vi "get mapped channels.vi"(7 "owner":string, 11 "engine configuration in":refnum<class "engine configuration.lvclass">) -> (1 "write channels":refnum<class "TBM channel.lvclass">[](array[class]), 2 "read channels":refnum<class "TBM channel.lvclass">[](array[class]), 3 "engine configuration out":refnum<class "engine configuration.lvclass">, 4 "paired read tag":refnum<class "tag descriptor.lvclass">[](array[class]), 6 "paired write tag":refnum<class "tag descriptor.lvclass">[](array[class]))   [LabVIEW 2013, in "engine configuration.lvclass"]
doc: "This function returns the list of the owner's read and write channels that have been mapped to tags."
uses:
  engine configuration.lvclass
  <vilib>/NI/Tag Bus Module Framework/channel/TBM channel.lvclass
  <vilib>/NI/Tag Bus/tag/tag descriptor.lvclass
  engine configuration.lvclass/engine configuration.ctl
  <vilib>/NI/Tag Bus/tag/tag descriptor.lvclass/tag descriptor.ctl
  <vilib>/NI/Tag Bus Module Framework/channel/channel classification.ctl
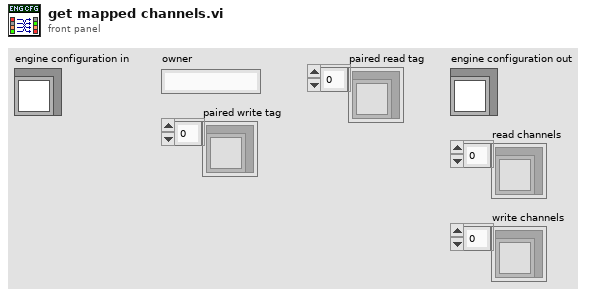
[diagram p1: front panel]
types:
  T1 = typedef "engine configuration.lvclass/module channel pairings.ctl" = cluster{"modules":string[], "channels":string[]}
  T2 = typedef "TBM channel.lvclass/channel classification.ctl" = enum16{"input data", "output data", "processing parameter", "processing result"}
  T3 = typedef "tag bus.lvlib/tag descriptor.lvclass/Data Type.ctl" = enum16{"Double", "Single", "I64", "I32", "I16", "I8", "U64", "U32", "U16", "U8", "Boolean", "String", "Array of Double", "Array of Single", "Array of I64", "Array of I32", "Array of I16", "Array of I8", "Array of U64", "Array of U32", "Array of U16", "Array of U8", "Array of Boolean", "Array of String"}
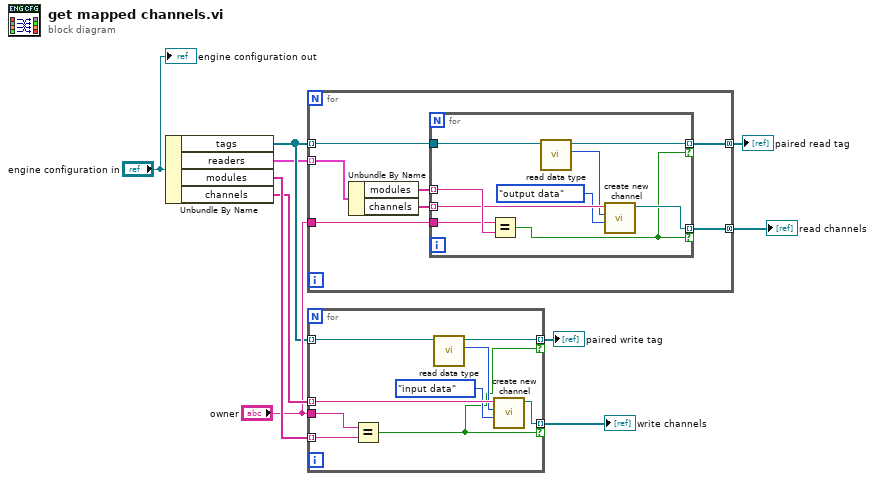
[diagram p0: block diagram]
diagram:
  n1 = Unbundle By Name("engine configuration in") -> ("tags"=w5:refnum<class "tag descriptor.lvclass">[], "readers"=w4:T1[], "modules"=w9:string[], "channels"=w8:string[])
  n2 = for {
    tunnel: "owner" -> [w17]
    tunnel: w5 -> [w16] mode=indexing
    tunnel: w4 -> [w15] mode=indexing
    tunnel: [w12] -> w3 mode=concatenating
    tunnel: [w11] -> w2 mode=concatenating
    n3 = Unbundle By Name(w15) -> ("modules"=w13:string[], "channels"=w14:string[])
    n4 = for {
      tunnel: w13 -> [w26] mode=indexing
      tunnel: w14 -> [w24] mode=indexing
      tunnel: w17 -> [w25]
      tunnel: [w22] -> w12 mode=indexing if=w18
      tunnel: w16 -> [w21]
      tunnel: [w19] -> w11 mode=indexing if=w18
      n5 = Equal?(x=w25, y=w26) -> (x = y?=w18:bool)
      n6 = call <vilib>:"read data type.vi"("system tag in"=w21) -> ("data type"=w20:T3, "system tag out"=w19:refnum<class "tag descriptor.lvclass">)  [unwired: 8 in, 1 out]
      n7 = call <vilib>:"create new channel.vi"("channel classification"=channel_classification."output data", "data type"=w20, "channel name"=w24) -> ("channel"=w22:refnum<class "TBM channel.lvclass">)  [unwired: 8 in]
    }
  }
  "read channels" <- w3
  "paired read tag" <- w2
  n8 = for {
    tunnel: w9 -> [w35] mode=indexing
    tunnel: w8 -> [w33] mode=indexing
    tunnel: "owner" -> [w34]
    tunnel: [w31] -> w7 mode=indexing if=w27
    tunnel: w5 -> [w30] mode=indexing
    tunnel: [w28] -> w1 mode=indexing if=w27
    n9 = Equal?(x=w34, y=w35) -> (x = y?=w27:bool)
    n10 = call <vilib>:"read data type.vi"("system tag in"=w30) -> ("data type"=w29:T3, "system tag out"=w28:refnum<class "tag descriptor.lvclass">)  [unwired: 8 in, 1 out]
    n11 = call <vilib>:"create new channel.vi"("channel classification"=channel_classification."input data", "data type"=w29, "channel name"=w33) -> ("channel"=w31:refnum<class "TBM channel.lvclass">)  [unwired: 8 in]
  }
  "write channels" <- w7
  "paired write tag" <- w1
  "engine configuration out" <- "engine configuration in"
